vi "Устройство умножения.vi"(1 "B":T2, 2 "A":T3) -> (0 "R":T1)   [LabVIEW 2017]
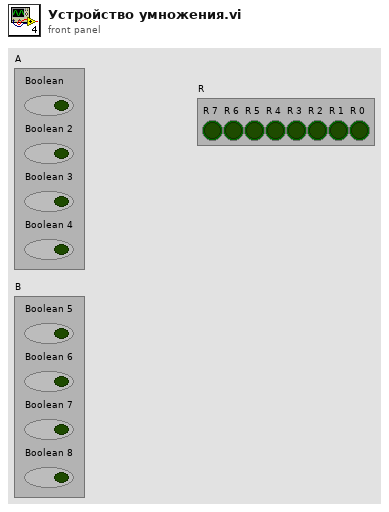
[diagram p1: front panel]
types:
  T1 = cluster{"R 7":bool, "R 6":bool, "R 5":bool, "R 4":bool, "R 3":bool, "R 2":bool, "R 1":bool, "R 0":bool}
  T2 = cluster{"Boolean 5":bool, "Boolean 6":bool, "Boolean 7":bool, "Boolean 8":bool}
  T3 = cluster{"Boolean":bool, "Boolean 2":bool, "Boolean 3":bool, "Boolean 4":bool}
  T4 = cluster{bool, "Boolean":bool, "Boolean 2":bool, "Boolean 3":bool}
  T5 = cluster{bool, "Boolean":bool, "Boolean 2":bool, "Boolean 3":bool, "Boolean 4":bool, "Boolean 4":bool, "Boolean 4":bool, bool}
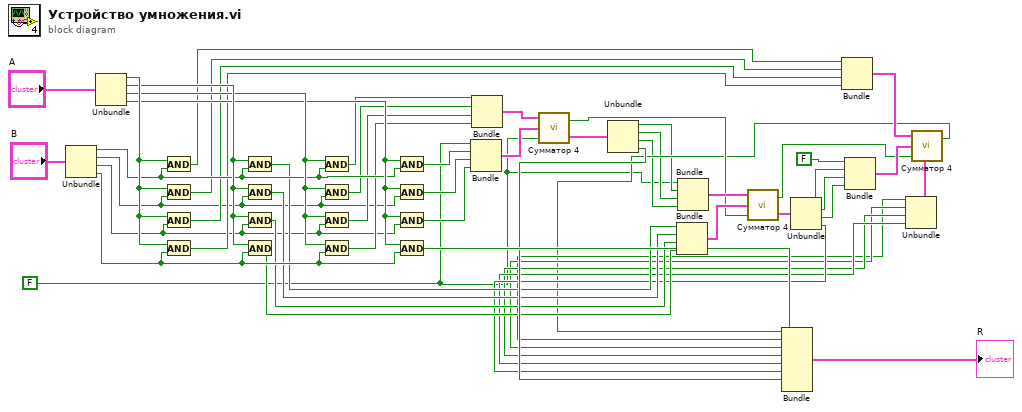
[diagram p0: block diagram]
diagram:
  w6 = FALSE
  n1 = Unbundle("B") -> ("Boolean 5"=w47:bool, "Boolean 6"=w13:bool, "Boolean 7"=w14:bool, "Boolean 8"=w46:bool)
  n2 = Unbundle("A") -> ("Boolean"=w51:bool, "Boolean 2"=w50:bool, "Boolean 3"=w49:bool, "Boolean 4"=w48:bool)
  n3 = And(x=w51, y=w47) -> (x .and. y?=w22:bool)
  n4 = And(x=w51, y=w13) -> (x .and. y?=w23:bool)
  n5 = And(x=w51, y=w14) -> (x .and. y?=w24:bool)
  n6 = And(x=w51, y=w46) -> (x .and. y?=w25:bool)
  n7 = And(x=w50, y=w47) -> (x .and. y?=w29:bool)
  n8 = And(x=w50, y=w13) -> (x .and. y?=w30:bool)
  n9 = And(x=w50, y=w14) -> (x .and. y?=w31:bool)
  n10 = And(x=w50, y=w46) -> (x .and. y?=w32:bool)
  n11 = And(x=w49, y=w47) -> (x .and. y?=w41:bool)
  n12 = And(x=w49, y=w13) -> (x .and. y?=w40:bool)
  n13 = And(x=w49, y=w14) -> (x .and. y?=w39:bool)
  n14 = And(x=w49, y=w46) -> (x .and. y?=w38:bool)
  n15 = And(x=w48, y=w47) -> (x .and. y?=w12:bool)
  n16 = And(x=w48, y=w13) -> (x .and. y?=w11:bool)
  n17 = And(x=w48, y=w14) -> (x .and. y?=w10:bool)
  n18 = And(x=w48, y=w46) -> (x .and. y?=w45:bool)
  n19 = Bundle(w6, w12, w11, w10) -> (w42:cluster{bool, bool, bool, bool})  [unwired: 1 in]
  n20 = Bundle(w41, w40, w39, w38) -> (w43:cluster{bool, bool, bool, bool})  [unwired: 1 in]
  n21 = call "Сумматор 4.vi"(2:w6, "B"=w42, "A"=w43) -> ("Summ"=w44:T3, 1:w33:bool)
  n22 = Unbundle(w44) -> ("Boolean"=w7:bool, "Boolean 2"=w8:bool, "Boolean 3"=w9:bool, "Boolean 4"=w37:bool)
  n23 = Bundle(w29, w30, w31, w32) -> (w34:cluster{bool, bool, bool, bool})  [unwired: 1 in]
  n24 = Bundle(w6, "Boolean"=w7, "Boolean 2"=w8, "Boolean 3"=w9) -> (w35:T4)  [unwired: 1 in]
  n25 = call "Сумматор 4.vi"(2:w33, "B"=w34, "A"=w35) -> ("Summ"=w36:T3, 1:w20:bool)
  n26 = Unbundle(w36) -> ("Boolean"=w3:bool, "Boolean 2"=w4:bool, "Boolean 3"=w5:bool, "Boolean 4"=w28:bool)
  n27 = Bundle(w22, w23, w24, w25) -> (w26:cluster{bool, bool, bool, bool})  [unwired: 1 in]
  n28 = Bundle(FALSE, "Boolean"=w3, "Boolean 2"=w4, "Boolean 3"=w5) -> (w21:T4)  [unwired: 1 in]
  n29 = call "Сумматор 4.vi"(2:w20, "B"=w21, "A"=w26) -> ("Summ"=w27:T3, 1:w15:bool)
  n30 = Unbundle(w27) -> ("Boolean"=w16:bool, "Boolean 2"=w17:bool, "Boolean 3"=w18:bool, "Boolean 4"=w19:bool)
  n31 = Bundle(w15, "Boolean"=w16, "Boolean 2"=w17, "Boolean 3"=w18, "Boolean 4"=w19, "Boolean 4"=w28, "Boolean 4"=w37, w45) -> (→"R":T5)  [unwired: 1 in]
